vi "Configure Voltage Trigger.vi"(8 "error in (no error)":errorcluster, 9 "Voltage Trigger Slope (0: Positive)":u16(ring) items=["Positive", "Negative"], 10 "Voltage Trigger Level (0 V)":dbl, 11 "VISA resource name":refnum<visa-resource-name>) -> (0 "error out":errorcluster, 3 "VISA resource name out":refnum<visa-resource-name>)   [LabVIEW 2021, in "Agilent N6900 N7900 Series.lvlib"]
doc: "Configures the settings necessary for a voltage-based trigger."
uses:
  <instrlib>/Agilent N6900 N7900 Series/Agilent N6900 N7900 Series.lvlib
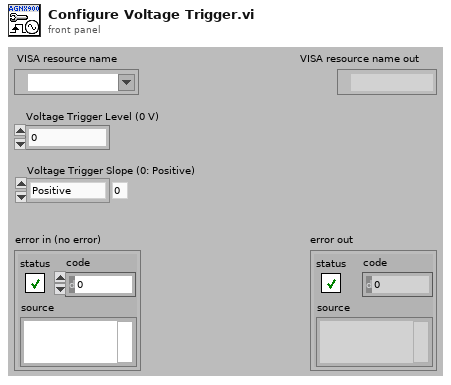
[diagram p1: front panel]
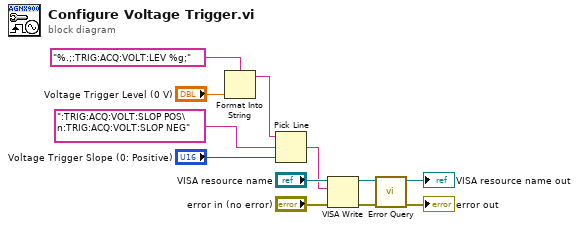
[diagram p0: block diagram]
diagram:
  n1 = Format Into String(format string="%.;:TRIG:ACQ:VOLT:LEV %g;", "Voltage Trigger Level (0 V)") -> (resulting string=w2:string)  [unwired: 2 in, 1 out]
  n2 = Pick Line(string ("")=w2, multi-line string=":TRIG:ACQ:VOLT:SLOP POS\n:TRIG:ACQ:VOLT:SLOP NEG", line index="Voltage Trigger Slope (0: Positive)") -> (output string=w6:string)
  n3 = VISA Write(VISA resource name="VISA resource name", write buffer=w6, error in (no error)="error in (no error)") -> (VISA resource name out=w9:refnum<visa-resource-name>, error out=w10:errorcluster)  [unwired: 1 out]
  n4 = call <instrlib>:"Error Query.vi"("error in (no error)"=w10, "VISA resource name"=w9) -> ("error out"=→"error out":errorcluster, "VISA resource name out"=→"VISA resource name out":refnum<visa-resource-name>)  [unwired: 6 in, 2 out]
